vi "GetDrive.vi"(8 "Error In":errorcluster) -> (0 "Error Out":errorcluster)   [LabVIEW 2020]
uses:
  <vilib>/Rock Robotics/WPI/ThirdParty/JAS_Junk/TrajLib/LinearFilter_ResetToValue.vi
  <vilib>/Rock Robotics/WPI/ThirdParty/JAS_Junk/TrajLib/LinearFilter_Calculate.vi
  <vilib>/Rock Robotics/WPI/ThirdParty/JAS_Junk/TrajLib/LinearFilter_MovingAverage.vi
  <vilib>/Rock Robotics/WPI/ThirdParty/JAS_Junk/TrajLib/LinearFilter_LowPassBW1.vi
  <vilib>/Rock Robotics/WPI/ThirdParty/JAS_Junk/TrajLib/LinearFilter_LowPassBW2.vi
  <vilib>/Rock Robotics/WPI/ThirdParty/JAS_Junk/TrajLib/LinearFilter_HighPassBW1.vi
  <vilib>/Rock Robotics/WPI/ThirdParty/JAS_Junk/TrajLib/LinearFilter_HighPassBW2.vi
  DriveGlobals.vi
  <vilib>/Rock Robotics/WPI/ThirdParty/JAS_Junk/TrajLib/Trajectory_Library.lvlib
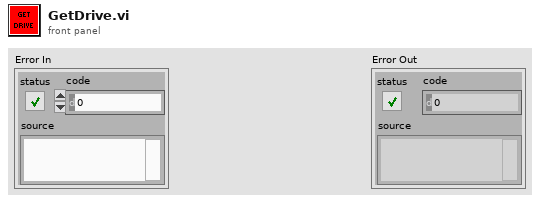
[diagram p1: front panel]
types:
  T1 = enum16{"Moving Average", "Low Pass 1st Order Butterworth", "Low Pass 2nd Order Butterworth", "High Pass 1st Order Butterworth", "High Pass 2nd Order Butterworth"}
  T2 = typedef "ADIS16470 Device Reference.ctl" = cluster{"DevStatus":errorcluster, "Hardware Config":T3, "Calibration Complete":refnum<notifier>, "Status Reference":refnum<data-value>, "Data Reference":refnum<data-value>, "Sychronous Process VI":T7, "Cmd FIFO":refnum<k33>, "Source":T8, "Data FIFO":refnum<k33>, "Calibration Time (ms)":u32, "Data Reference":refnum<data-value>}
  T3 = typedef "ADIS16470 Hardware Configuration.ctl" = cluster{"SPI Clock Rate (Hz)":dbl, "IMU SPI Mode (3)":T4, "IMU Reset Pin":T5, "IMU SPI Bus":T6, "IMU Data Ready Pin":T5, "Stall Config":cluster{"Pow2BytesPerRead":u8, "StallTicks":u16, "CsToSclkTicks":u8}}
  T4 = typedef "WPI_SPIMode.ctl" = enum16{"Mode 0 (Clk Idle Low,Sample on Leading)", "Mode 1 (Clk Idle Low,Sample on Trailing)", "Mode 2 (Clk Idle High,Sample on Leading)", "Mode 3 (Clk Idle High,Sample on Trailing)"}
  T5 = typedef "FPGA_DIOChannel.ctl" = enum8{"DIO 0", "DIO 1", "DIO 2", "DIO 3", "DIO 4", "DIO 5", "DIO 6", "DIO 7", "DIO 8", "DIO 9", "DIO MXP 0", "DIO MXP 1", "DIO MXP 2", "DIO MXP 3", "DIO MXP 4", "DIO MXP 5", "DIO MXP 6", "DIO MXP 7", "DIO MXP 8", "DIO MXP 9", "DIO MXP 10", "DIO MXP 11", "DIO MXP 12", "DIO MXP 13", "DIO MXP 14", "DIO MXP 15", "SPI Port CS1", "SPI Port CS2", "SPI Port CS3", "SPI Port MISO", "SPI Port MOSI", "Invalid"}
  T6 = typedef "spi_bus.ctl" = enum16{"SPI On-Board, CS0", "SPI On-Board, CS1", "SPI On-Board, CS2", "SPI On-Board, CS3", "SPI MXP", "Invalid"}
  T7 = typedef "ADIS16470 Process.ctl" = refnum<vi>
  T8 = typedef "FPGA_CounterEncoderSourceConvertionLVSourceType.ctl" = cluster{"DevStatus":errorcluster, "AnalogTriggerMode?":bool, "DigitalMode":cluster{"DIO Channel":T9}, "AnalogTriggerMode":cluster{"AnalogTriggerIndex":T10, "OutputType":T11}}
  T9 = typedef "FPGA_DIODigitalSourceChannel.ctl" = enum8{"DIO 0", "DIO 1", "DIO 2", "DIO 3", "DIO 4", "DIO 5", "DIO 6", "DIO 7", "DIO 8", "DIO 9", "DIO MXP 0", "DIO MXP 1", "DIO MXP 2", "DIO MXP 3", "DIO MXP 4", "DIO MXP 5", "DIO MXP 6", "DIO MXP 7", "DIO MXP 8", "DIO MXP 9", "DIO MXP 10", "DIO MXP 11", "DIO MXP 12", "DIO MXP 13", "DIO MXP 14", "DIO MXP 15", "SPI Port CS1", "SPI Port CS2", "SPI Port CS3", "SPI Port MISO", "SPI Port MOSI", "Disabled"}
  T10 = typedef "FPGA_AnalogTriggerIndex.ctl" = enum8{"Trig 0", "Trig 1", "Trig 2", "Trig 3", "Trig 4", "Trig 5", "Trig 6", "Trig 7", "Invalid"}
  T11 = typedef "FPGA_AnalogTriggerOutType.ctl" = enum16{"InWindow", "TriggerState", "Rising", "Falling"}
  T12 = typedef "ADIS16470 Status.ctl" = cluster{"Calibrated?":bool, "IMU Detected?":bool}
  T13 = typedef "WPI_EncoderDevRef.ctl" = cluster{"DevStatus":errorcluster, "EncoderIndex":T14, "CounterIndex":T15, "DistancePerCount":dbl, "Decoding Type":T16}
  T14 = typedef "FPGA_EncoderIdx.ctl" = enum8{"Enc 0", "Enc 1", "Enc 2", "Enc 3", "Enc 4", "Enc 5", "Enc 6", "Enc 7", "Invalid"}
  T15 = typedef "FPGA_CounterCtrSystemIndex.ctl" = enum8{"Ctr 0", "Ctr 1", "Ctr 2", "Ctr 3", "Ctr 4", "Ctr 5", "Ctr 6", "Ctr 7", "Invalid"}
  T16 = typedef "WPI_EncoderType.ctl" = enum16{"1x", "2x", "4x"}
  T17 = typedef "ADIS16470 Data.ctl" = cluster{"XAngle":dbl, "YAngle":dbl, "ZAngle":dbl}
  T18 = typedef "WPI_CounterDevRef.ctl" = cluster{"DevStatus":errorcluster, "CntIndex":T15}
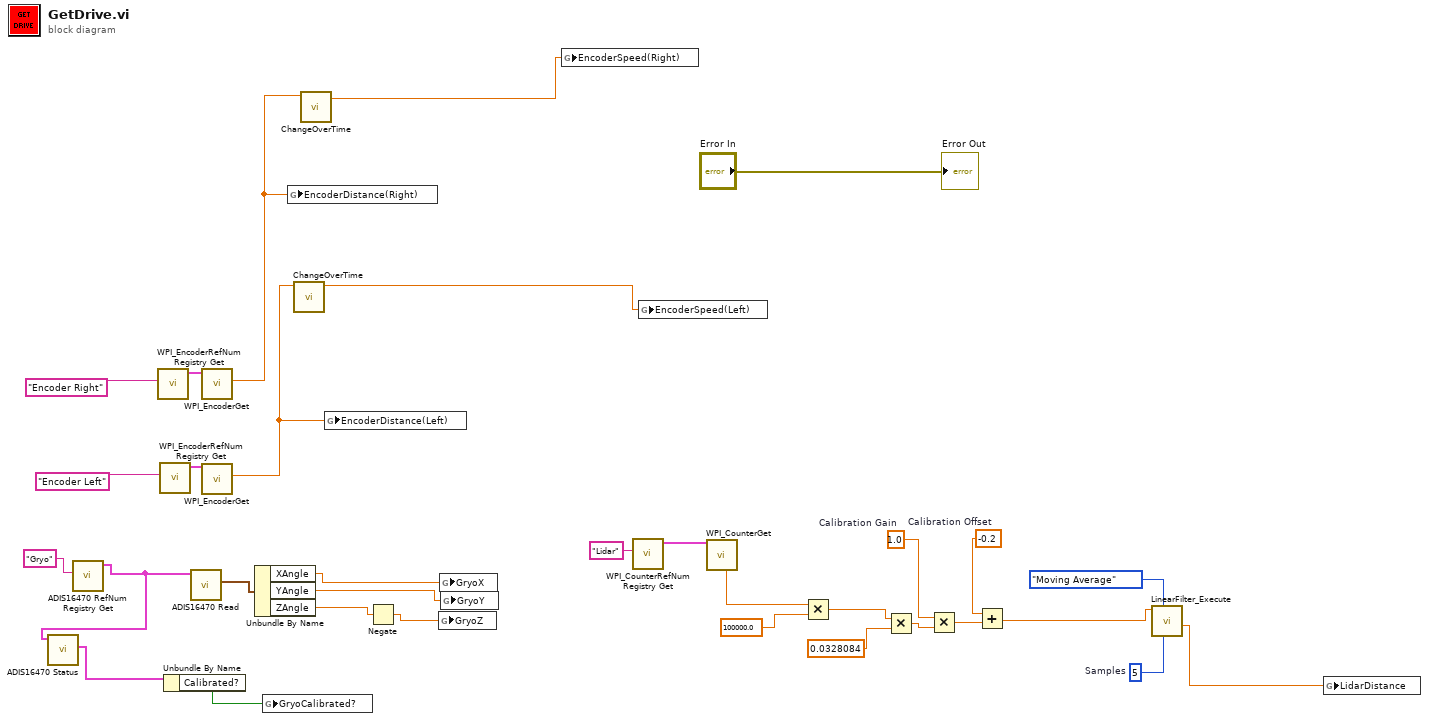
[diagram p0: block diagram]
diagram:
  w10 = 5  # Samples
  w13 = -0.2  # Calibration Offset
  w14 = 1.0  # Calibration Gain
  n1 = call <vilib>:"ADIS16470 RefNum Registry Get.vi"("refnum name"="Gryo") -> ("ADIS16470DevRef out"=w3:T2)  [unwired: 9 in, 1 out]
  n2 = call <vilib>:"ADIS16470 Status.vi"("ADIS16470DevRef"=w3) -> ("ADIS16470 Status"=w4:T12)  [unwired: 8 in, 2 out]
  n3 = call <vilib>:"WPI_EncoderRefNum Registry Get.vi"("refnum name"="Encoder Right") -> ("EncoderDevRef"=w29:T13)  [unwired: 9 in, 1 out]
  n4 = call <vilib>:"WPI_EncoderRefNum Registry Get.vi"("refnum name"="Encoder Left") -> ("EncoderDevRef"=w30:T13)  [unwired: 9 in, 1 out]
  n5 = Unbundle By Name(w4) -> ("Calibrated?"=w21:bool)
  n6 = call <vilib>:"ADIS16470 Read.vi"("ADIS16470DevRef"=w3) -> ("ADIS16470 Value"=w5:T17)  [unwired: 7 in, 3 out]
  n7 = call <vilib>:"WPI_EncoderGet.vi"("EncoderDevRef"=w29) -> ("Distance"=w27:dbl)  [unwired: 5 in, 5 out]
  n8 = call <vilib>:"WPI_EncoderGet.vi"("EncoderDevRef"=w30) -> ("Distance"=w26:dbl)  [unwired: 5 in, 5 out]
  n9 = Unbundle By Name(w5) -> ("XAngle"=w23:dbl, "YAngle"=w22:dbl, "ZAngle"=w1:dbl)
  n10 = global write "DriveGlobals.vi" "GryoCalibrated?"(w21) -> ()
  n11 = global write "DriveGlobals.vi" "EncoderDistance(Right)"(w27) -> ()
  n12 = call "ChangeOverTime.vi"("InputNum"=w26) -> ("ChangeOverTime"=w24:dbl)  [unwired: 10 in]
  n13 = call "ChangeOverTime.vi"("InputNum"=w27) -> ("ChangeOverTime"=w28:dbl)  [unwired: 10 in]
  n14 = global write "DriveGlobals.vi" "EncoderDistance(Left)"(w26) -> ()
  n15 = Negate(x=w1) -> (-x=w2:dbl)
  n16 = global write "DriveGlobals.vi" "GryoZ"(w2) -> ()
  n17 = global write "DriveGlobals.vi" "GryoX"(w23) -> ()
  n18 = global write "DriveGlobals.vi" "GryoY"(w22) -> ()
  n19 = global write "DriveGlobals.vi" "EncoderSpeed(Right)"(w28) -> ()
  n20 = call <vilib>:"WPI_CounterRefNum Registry Get.vi"("refnum name"="Lidar") -> ("CounterDevRef"=w19:T18)  [unwired: 9 in, 1 out]
  n21 = global write "DriveGlobals.vi" "EncoderSpeed(Left)"(w24) -> ()
  n22 = call <vilib>:"WPI_CounterGet.vi"("CounterDevRef in"=w19) -> ("Period (sec)"=w17:dbl)  [unwired: 5 in, 5 out]
  n23 = Multiply(x=w17, y=100000.0) -> (x*y=w18:dbl)
  n24 = Multiply(x=w18, y=0.0328084) -> (x*y=w12:dbl)
  n25 = Multiply(x=w14, y=w12) -> (x*y=w11:dbl)
  n26 = Add(x=w13, y=w11) -> (x+y=w8:dbl)
  n27 = call <vilib>:"LinearFilter_Execute.vi"("Samples"=w10, "Filter Type"=T1."Moving Average", "Input"=w8) -> ("Output"=w7:dbl)  [unwired: 7 in, 1 out]
  n28 = global write "DriveGlobals.vi" "LidarDistance"(w7) -> ()
  "Error Out" <- "Error In"
